vi "Register gRPC Messages.vi"(8 "error in (no error)":errorcluster, 11 "Template Server in":refnum<class "Data Marshal Server.lvclass">) -> (0 "error out":errorcluster, 3 "Template Server out":refnum<class "Data Marshal Server.lvclass">)   [LabVIEW 2019, in "Data Marshal Server.lvlib" / "Data Marshal Server.lvclass"]
uses:
  Data Marshal Server.lvclass
  gRPC lvSupport/Server API/typeDefs/Message Metadata.ctl
  gRPC lvSupport/Server API/typeDefs/Message Element Metadata.ctl
  gRPC lvSupport/Server API/typeDefs/Message Element Type.ctl
  Data Marshal Server.lvclass/Data Marshal Server.ctl
  gRPC lvSupport/gprc-lvsupport.lvlib
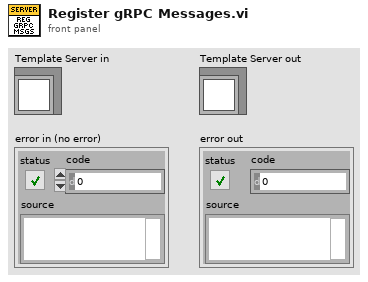
[diagram p1: front panel]
types:
  T1 = typedef "Data Marshal Server.lvlib/gprc-lvsupport.lvlib/Message Metadata.ctl" = cluster{"Name":string, "Elements":T2[]}
  T2 = typedef "Data Marshal Server.lvlib/gprc-lvsupport.lvlib/Message Element Metadata.ctl" = cluster{"Embedded Message Name":string, "Protobuf Index":i32, "MessageElementType":T3, "Repeated":bool}
  T3 = typedef "Data Marshal Server.lvlib/gprc-lvsupport.lvlib/Message Element Type.ctl" = enum32{"Int32Value", "FloatValue", "DoubleValue", "BoolValue", "StringValue", "MessageValue", "Int64Value", "UInt32Value", "UInt64Value", "EnumValue"}
  T4 = typedef "Data Marshal Server.lvlib/gprc-lvsupport.lvlib/grpcId.ctl" = u64
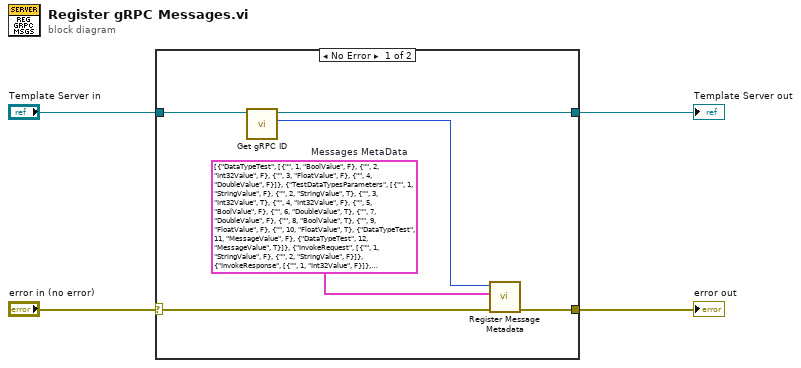
[diagram p0: block diagram]
diagram:
  n1 = case shown="No Error" "error in (no error)" {
    selector: "error in (no error)" -> [w5 w12]
    tunnel: [w10 w11] -> w4
    tunnel: [w9 w12] -> w3
    tunnel: "Template Server in" -> [w7 w11]
    frame No Error {
      w6 = T1[] [{"Name"="DataTypeTest", "Elements"=[{"Embedded Message Name"="", "Protobuf Index"=1, "MessageElementType"=enum."BoolValue", "Repeated"=FALSE}, {"Embedded Message Name"="", "Protobuf Index"=2, "MessageElementType"=enum."Int32Value", "Repeated"=FALSE}, {"Embedded Message Name"="", "Protobuf Index"=3, "MessageElementType"=enum."FloatValue", "Repeated"=FALSE}, {"Embedded Message Name"="", "Protobuf Index"=4, "MessageElementType"=enum."DoubleValue", "Repeated"=FALSE}]}, {"Name"="TestDataTypesParameters", "Elements"=[{"Embedded Message Name"="", "Protobuf Index"=1, "MessageElementType"=enum."StringValue", "Repeated"=FALSE}, {"Embedded Message Name"="", "Protobuf Index"=2, "MessageElementType"=enum."StringValue", "Repeated"=TRUE}, {"Embedded Message Name"="", "Protobuf Index"=3, "MessageElementType"=enum."Int32Value", "Repeated"=TRUE}, {"Embedded Message Name"="", "Protobuf Index"=4, "MessageElementType"=enum."Int32Value", "Repeated"=FALSE}, {"Embedded Message Name"="", "Protobuf Index"=5, "MessageElementType"=enum."BoolValue", "Repeated"=FALSE}, {"Embedded Message Name"="", "Protobuf Index"=6, "MessageElementType"=enum."DoubleValue", "Repeated"=TRUE}, {"Embedded Message Name"="", "Protobuf Index"=7, "MessageElementType"=enum."DoubleValue", "Repeated"=FALSE}, {"Embedded Message Name"="", "Protobuf Index"=8, "MessageElementType"=enum."BoolValue", "Repeated"=TRUE}, {"Embedded Message Name"="", "Protobuf Index"=9, "MessageElementType"=enum."FloatValue", "Repeated"=FALSE}, {"Embedded Message Name"="", "Protobuf Index"=10, "MessageElementType"=enum."FloatValue", "Repeated"=TRUE}, {"Embedded Message Name"="DataTypeTest", "Protobuf Index"=11, "MessageElementType"=enum."MessageValue", "Repeated"=FALSE}, {"Embedded Message Name"="DataTypeTest", "Protobuf Index"=12, "MessageElementType"=enum."MessageValue", "Repeated"=TRUE}]}, {"Name"="InvokeRequest", "Elements"=[{"Embedded Message Name"="", "Protobuf Index"=1, "MessageElementType"=enum."StringValue", "Repeated"=FALSE}, {"Embedded Message Name"="", "Protobuf Index"=2, "MessageElementType"=enum."StringValue", "Repeated"=FALSE}]}, {"Name"="InvokeResponse", "Elements"=[{"Embedded Message Name"="", "Protobuf Index"=1, "MessageElementType"=enum."Int32Value", "Repeated"=FALSE}]}, {"Name"="QueryRequest", "Elements"=[{"Embedded Message Name"="", "Protobuf Index"=1, "MessageElementType"=enum."StringValue", "Repeated"=FALSE}]}, {"Name"="QueryResponse", "Elements"=[{"Embedded Message Name"="", "Protobuf Index"=1, "MessageElementType"=enum."StringValue", "Repeated"=FALSE}, {"Embedded Message Name"="", "Protobuf Index"=2, "MessageElementType"=enum."Int32Value", "Repeated"=FALSE}]}, {"Name"="RegistrationRequest", "Elements"=[{"Embedded Message Name"="", "Protobuf Index"=1, "MessageElementType"=enum."StringValue", "Repeated"=FALSE}]}, {"Name"="ServerEvent", "Elements"=[{"Embedded Message Name"="", "Protobuf Index"=1, "MessageElementType"=enum."StringValue", "Repeated"=FALSE}, {"Embedded Message Name"="", "Protobuf Index"=2, "MessageElementType"=enum."Int32Value", "Repeated"=FALSE}, {"Embedded Message Name"="", "Protobuf Index"=3, "MessageElementType"=enum."Int32Value", "Repeated"=FALSE}]}]  # Messages MetaData
      n2 = call "Get gRPC ID.vi"("OOP Server in"=w7) -> ("gRPC ID"=w8:T4, "OOP Server out"=w10:refnum<class "Data Marshal Server.lvclass">)  [unwired: 9 in]
      n3 = call "Register Message Metadata.vi"("error in (no error)"=w5, "Messages"=w6, "gRPCid"=w8) -> ("error out"=w9:errorcluster)  [unwired: 7 in, 1 out]
    }
    frame Error {
    }
  }
  "Template Server out" <- w4
  "error out" <- w3
